vi "Read write file if changed.vi"(8 "error in (no error)":errorcluster, 11 "INIFileClass in":refnum<class "INIFileClass.lvclass">) -> (0 "error out":errorcluster, 2 "write file if changed":bool=TRUE, 3 "INIFileClass out":refnum<class "INIFileClass.lvclass">)   [LabVIEW 2013, in "INIFileClass.lvclass"]
uses:
  INIFileClass.lvclass
  INIFileClass.lvclass/INIFileClass.ctl
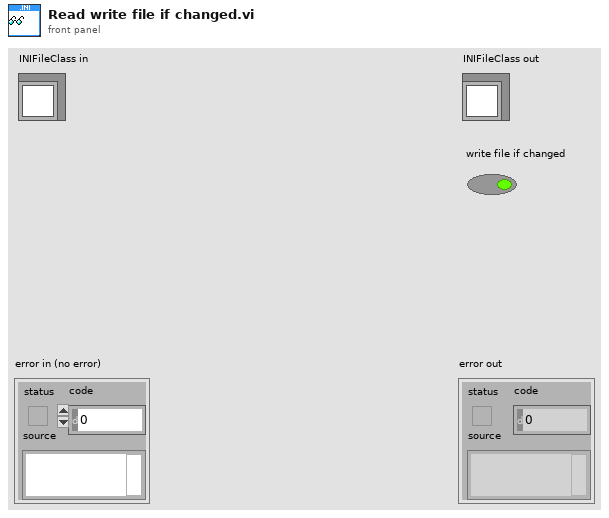
[diagram p1: front panel]
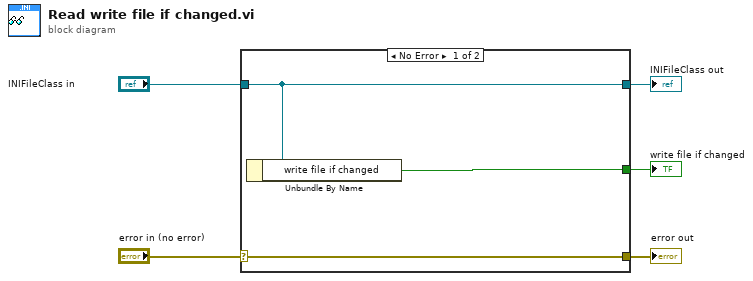
[diagram p0: block diagram]
diagram:
  n1 = case shown="No Error" "error in (no error)" {
    selector: "error in (no error)" -> [w8 w9]
    tunnel: [w8 w9] -> w4
    tunnel: [w7 w10] -> w2
    tunnel: "INIFileClass in" -> [w7 w10]
    tunnel: [w6 _] -> w1
    frame No Error {
      n2 = Unbundle By Name(w7) -> ("write file if changed"=w6:bool)
    }
    frame Error {
    }
  }
  "error out" <- w4
  "INIFileClass out" <- w2
  "write file if changed" <- w1
